vi "Delete Math Expression.vi"(7 "Expression Name (\"\")":string="\"\"", 8 "error in (no error)":errorcluster, 9 "Deletion Mode (1: Delete All)":i32(ring)=1 items=["Delete One", "Delete All"], 10 "Channel (0: Channel 1)":i32(ring) items=["Channel 1", "Channel 2"], 11 "VISA resource name":refnum<visa-resource-name>) -> (0 "error out":errorcluster, 3 "VISA resource name out":refnum<visa-resource-name>)   [LabVIEW 2023, in "Agilent B2900 Series.lvlib"]
doc: "Delete user-defined math expression(s)."
uses:
  Agilent B2900 Series.lvlib
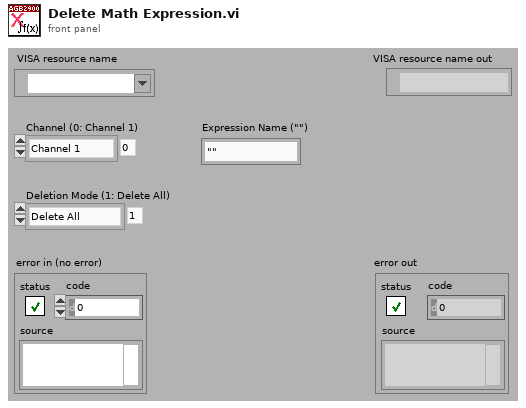
[diagram p1: front panel]
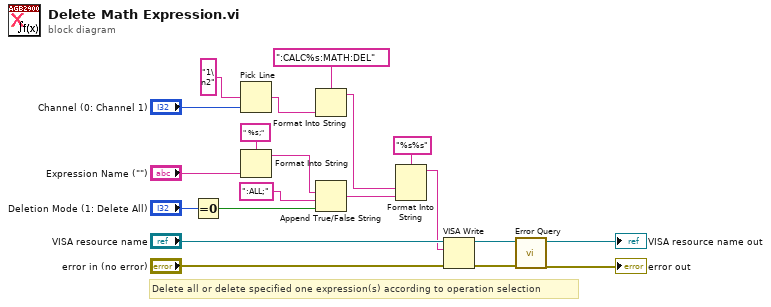
[diagram p0: block diagram]
diagram:
  # "Delete all or delete specified one expression(s) according to operation selection"
  n1 = Equal To 0?(x="Deletion Mode (1: Delete All)") -> (x = 0?=w5:bool)
  n2 = Pick Line(multi-line string="1\n2" ("string (\"\")"), line index="Channel (0: Channel 1)") -> (output string=w11:string)  [unwired: 1 in]
  n3 = Format Into String(format string=" %s;", "Expression Name (\"\")") -> (resulting string=w3:string)  [unwired: 2 in, 1 out]
  n4 = Format Into String(format string=":CALC%s:MATH:DEL", w11) -> (resulting string=w9:string)  [unwired: 2 in, 1 out]
  n5 = Append True/False String(1:w5, 2:":ALL;", 3:w3) -> (0:w1:string)  [unwired: 1 in]
  n6 = Format Into String(format string="%s%s", w9, w1) -> (resulting string=w8:string)  [unwired: 2 in, 1 out]
  n7 = VISA Write(VISA resource name="VISA resource name", write buffer=w8, error in (no error)="error in (no error)") -> (VISA resource name out=w18:refnum<visa-resource-name>, error out=w17:errorcluster)  [unwired: 1 out]
  n8 = call "Error Query.vi"("error in (no error)"=w17, "VISA resource name"=w18) -> ("error out"=→"error out":errorcluster, "VISA resource name out"=→"VISA resource name out":refnum<visa-resource-name>)  [unwired: 6 in, 2 out]
